vi "GSP_GetNextToken.vi"(0 "Input string":string) -> (1 "Token":string, 2 "Output string":string)   [LabVIEW 2015]
doc: "Get the next token from a string.\nReturns the token and the string without\nthe token."
panel:
  out "Offset index":i32
  out "Token length":i32
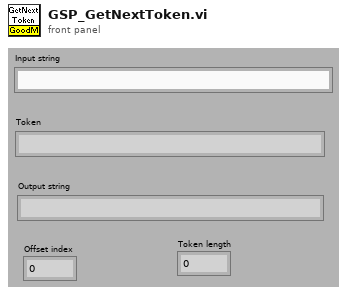
[diagram p1: front panel]
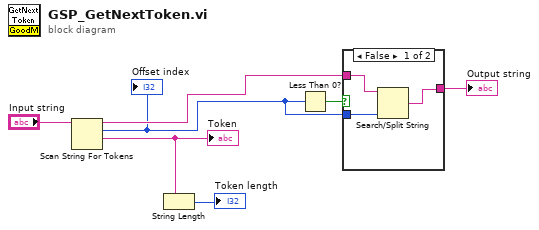
[diagram p0: block diagram]
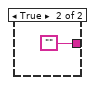
[diagram p2: hidden frame]
diagram:
  n1 = Scan String For Tokens(9:"Input string") -> (1:w6:string, 2:w1:i32, 3:w3:string)  [unwired: 5 in, 1 out]
  "Token" <- w6
  "Offset index" <- w1
  n2 = String Length(string=w6) -> (length=→"Token length":i32)
  n3 = Less Than 0?(x=w1) -> (x < 0?=w4:bool)
  n4 = case shown="False" w4 {
    tunnel: w3 -> [w9 _]
    tunnel: [w8 ""] -> w2
    tunnel: w1 -> [w10 _]
    frame False {
      n5 = Search/Split String(string=w9, offset (0)=w10) -> (match + rest of string=w8:string)  [unwired: 1 in, 2 out]
    }
    frame True {
    }
  }
  "Output string" <- w2
